vi "str.vi"(8 "error in (no error)":errorcluster, 11 "TestCase in":refnum<class "TestCase.lvclass">) -> (0 "error out":errorcluster, 2 "string":string, 3 "TestCase out":refnum<class "TestCase.lvclass">)   [LabVIEW 2013, in "TestCase.lvclass"]
doc: "method name[tab]class name"
uses:
  TestCase.lvclass
  TestCase.lvclass/TestCase.ctl
  Libraries/VITesterUtilities.lvlib
panel:
  # "JKI VI Tester for LabVIEW\nhttp://jkisoft.com/vi-tester\nCopyright (C) 2007-2009, JKI <info@jkisoft.com>\nALL RIGHTS RESERVED"
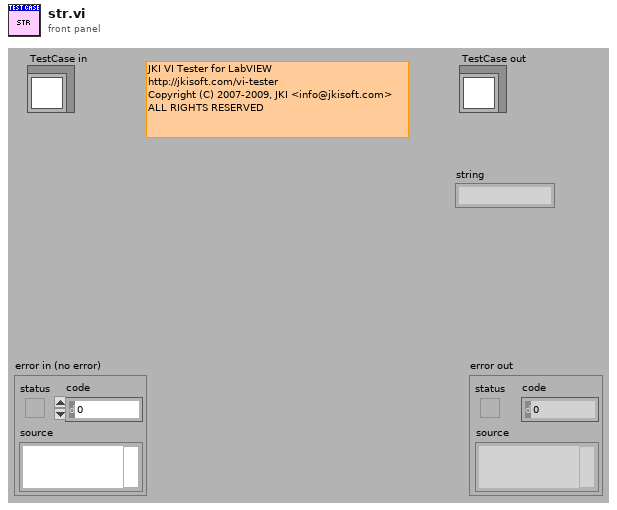
[diagram p1: front panel]
types:
  T1 = typedef "TestCase.lvclass/testMethodName.ctl" = string
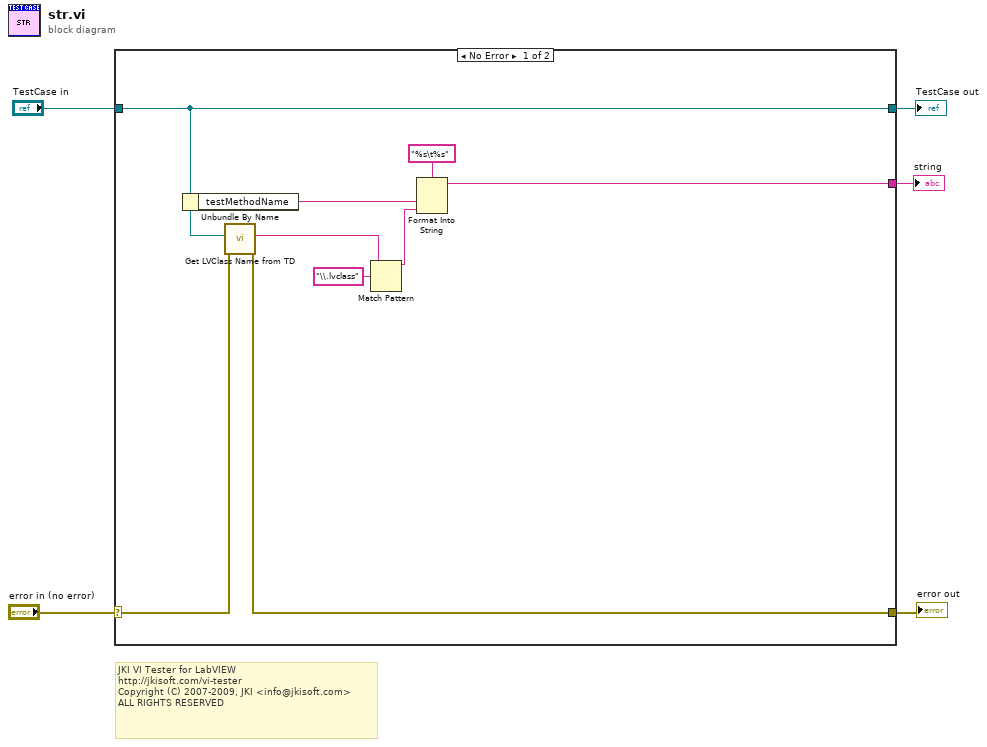
[diagram p0: block diagram]
diagram:
  # "JKI VI Tester for LabVIEW\nhttp://jkisoft.com/vi-tester\nCopyright (C) 2007-2009, JKI <info@jkisoft.com>\nALL RIGHTS RESERVED"
  n1 = case shown="No Error" "error in (no error)" {
    selector: "error in (no error)" -> [w7 w16]
    tunnel: [w6 w16] -> w4
    tunnel: [w13 w15] -> w2
    tunnel: "TestCase in" -> [w13 w15]
    tunnel: [w8 _] -> w1
    frame No Error {
      n2 = Unbundle By Name(w13) -> ("testMethodName"=w14:T1)
      n3 = call "Get LVClass Name from TD.vi"("error in"=w7, "Variant"=w13) -> ("error out"=w6:errorcluster, "LVClass Name"=w10:string)  [unwired: 8 in]
      n4 = Match Pattern(string=w10, regular expression="\\.lvclass") -> (before substring=w9:string)  [unwired: 1 in, 3 out]
      n5 = Format Into String(format string="%s\t%s", w14, w9) -> (resulting string=w8:string)  [unwired: 2 in, 1 out]
    }
    frame Error {
    }
  }
  "error out" <- w4
  "TestCase out" <- w2
  "string" <- w1
